vi "DIGIT_5122_Run_Write_Stop.vi"(8 "error in (no error)":errorcluster, 10 "QMH ICR Cluster":T1, 11 "instrument handle in":refnum<k15>) -> (0 "error out":errorcluster, 3 "dataset":i16[][](array[numeric]))   [LabVIEW 2024]
doc: "This VI is a standalone test for the PXIe-5122 digitizer.\n\nIf software trigger is used, the acquisition starts immediately reading channel 0.\nIf an external trigger is used, please connect a TTL trigger to the EXT TRIG connector in front panel of the PXIe-5122 board."
uses:
  controls/QMH_ICR_Cluster.ctl
  controls/HARDWARE_Resources.ctl
  controls/PROCESSING_Inputs.ctl
  controls/LOOPS_Inputs.ctl
  controls/OPO_Inputs.ctl
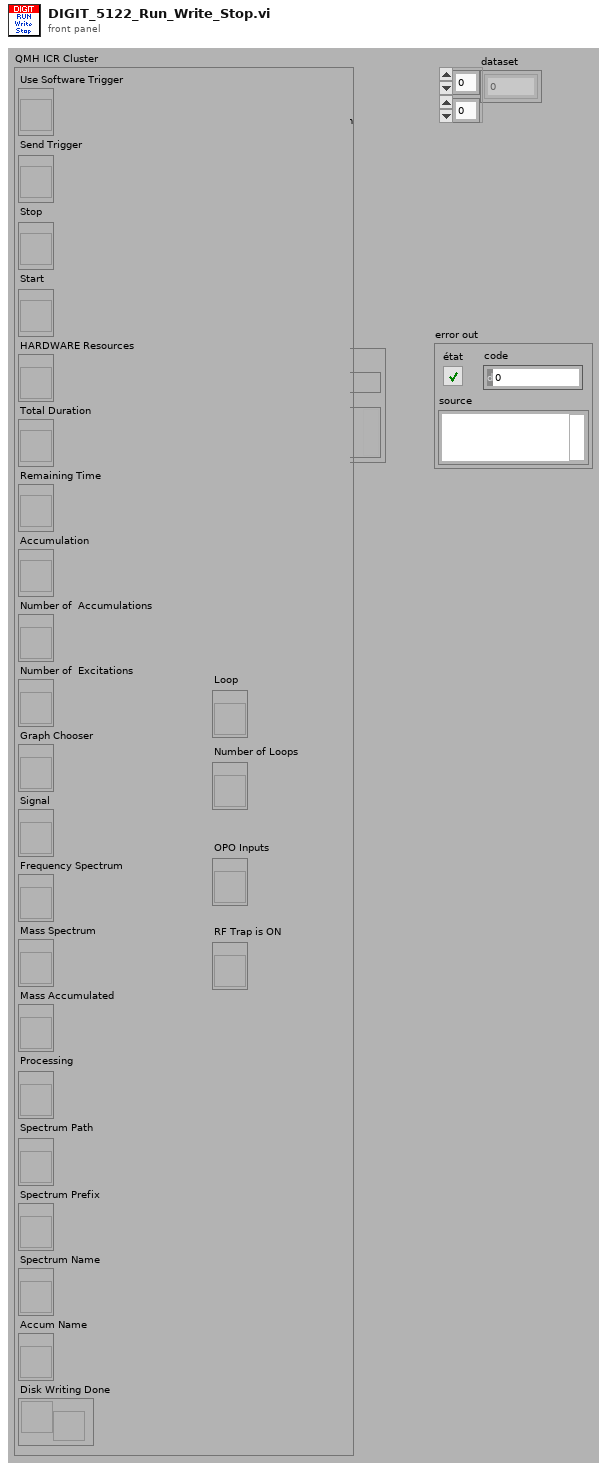
[diagram p1: front panel]
types:
  T1 = typedef "QMH_ICR_Cluster.ctl" = cluster{"Use Software Trigger":refnum<vi>, "Send Trigger":refnum<vi>, "Stop":refnum<vi>, "Start":refnum<vi>, "HARDWARE Resources":refnum<vi>, "Total Duration":refnum<vi>, "Remaining Time":refnum<vi>, "Accumulation":refnum<vi>, "Number of  Accumulations":refnum<vi>, "Number of  Excitations":refnum<vi>, "Graph Chooser":refnum<vi>, "Signal":refnum<vi>, "Frequency Spectrum":refnum<vi>, "Mass Spectrum":refnum<vi>, "Mass Accumulated":refnum<vi>, "Processing":refnum<vi>, "Spectrum Path":refnum<vi>, "Spectrum Prefix":refnum<vi>, "Spectrum Name":refnum<vi>, "Accum Name":refnum<vi>, "Disk Writing Done":refnum<notifier>, "Loop":refnum<vi>, "Number of Loops":refnum<vi>, "OPO Inputs":refnum<vi>, "RF Trap is ON":refnum<vi>}
  T2 = cluster{"actualSamples":i32, "absoluteInitialX":dbl, "relativeInitialX":dbl, "xIncrement":dbl, "offset":dbl, "gain":dbl, "reserved1":dbl, "reserved2":dbl}[]
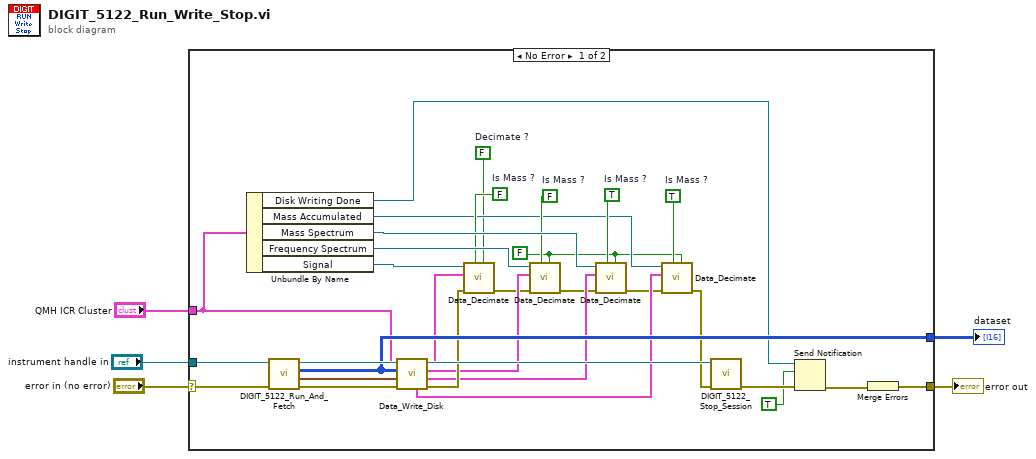
[diagram p0: block diagram]
diagram:
  n1 = case shown="No Error" "error in (no error)" {
    selector: "error in (no error)" -> [w33 w37]
    tunnel: [w34 w37] -> w4
    tunnel: [w28 _] -> w3
    tunnel: "QMH ICR Cluster" -> [w11 _]
    tunnel: "instrument handle in" -> [w32 _]
    frame No Error {
      w6 = FALSE
      w7 = FALSE  # Decimate ?
      w16 = TRUE  # Is Mass ?
      w20 = TRUE  # Is Mass ?
      w21 = FALSE  # Is Mass ?
      w22 = FALSE  # Is Mass ?
      n2 = Unbundle By Name(w11) -> ("Disk Writing Done"=w13:refnum<notifier>, "Mass Accumulated"=w17:refnum<vi>, "Mass Spectrum"=w25:refnum<vi>, "Frequency Spectrum"=w31:refnum<vi>, "Signal"=w30:refnum<vi>)
      n3 = call "DIGIT_5122_Run_And_Fetch.vi"("error in (no error)"=w33, "instrument handle"=w32) -> ("error out"=w36:errorcluster, "wfm info"=w29:T2, "dataset"=w28:i16[][], "instrument handle out"=w35:refnum<k15>)  [unwired: 6 in]
      n4 = call "Data_Write_Disk.vi"("error in (no error)"=w36, "wfm info"=w29, "dataset"=w28, "QMH ICR Cluster"=w11) -> ("error out"=w27:errorcluster, "Mass Spectrum"=w23:cluster{sgl[], sgl[]}[], "Frequency Spectrum"=w26:cluster{sgl[], sgl[]}[], "Dataset Signal"=w24:cluster{sgl[], sgl[]}[], "Mass Accumulated"=w18:cluster{"mass":sgl[], sgl[]}[])  [unwired: 3 in]
      n5 = call "Data_Decimate.vi"("Decimate ?"=w7, "Is Mass ?"=w22, "error in (no error)"=w27, "Dataset"=w24, "GraphXY"=w30) -> ("error out"=w10:errorcluster)  [unwired: 6 in]
      n6 = call "Data_Decimate.vi"("Decimate ?"=w6, "Is Mass ?"=w21, "error in (no error)"=w10, "Dataset"=w26, "GraphXY"=w31) -> ("error out"=w8:errorcluster)  [unwired: 6 in]
      n7 = call "Data_Decimate.vi"("Decimate ?"=w6, "Is Mass ?"=w20, "error in (no error)"=w8, "Dataset"=w23, "GraphXY"=w25) -> ("error out"=w9:errorcluster)  [unwired: 6 in]
      n8 = call "Data_Decimate.vi"("Decimate ?"=w6, "Is Mass ?"=w16, "error in (no error)"=w9, "Dataset"=w18, "GraphXY"=w17) -> ("error out"=w19:errorcluster)  [unwired: 6 in]
      n9 = call "DIGIT_5122_Stop_Session.vi"("error in (no error)"=w19, "instrument handle"=w35) -> ("error out"=w15:errorcluster)  [unwired: 9 in]
      n10 = Send Notification(notification=TRUE, notifier=w13, error in (no error)=w15) -> (error out=w14:errorcluster)  [unwired: 1 out]
      n11 = Merge Errors(w14) -> (w34:errorcluster)
    }
    frame Error {
    }
  }
  "error out" <- w4
  "dataset" <- w3
